vi "Log Monitor State Helper.vi"(6 "Laser ON?":bool, 7 "State Info":string, 8 "error in (no error)":errorcluster, 9 "Monitor":bool, 10 "STATUS.Ready":bool, 11 "EventLog in":refnum<class "EventLog.lvclass">) -> (0 "error out":errorcluster, 3 "EventLog out":refnum<class "EventLog.lvclass">)   [LabVIEW 2015, in "Tool Module.lvlib"]
uses:
  Tool Module.lvlib
  Event Logger Library/Event Log/EventLog.lvclass
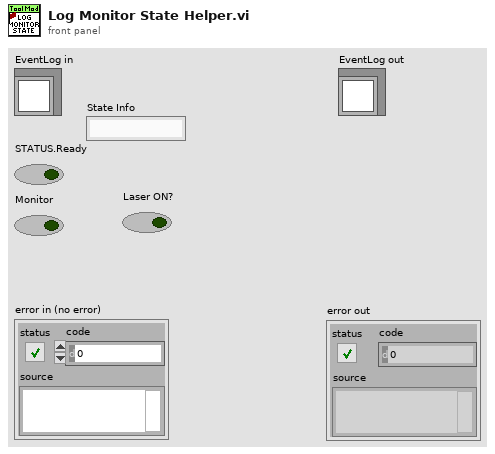
[diagram p1: front panel]
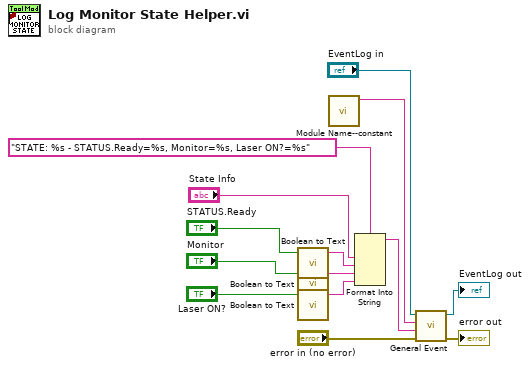
[diagram p0: block diagram]
diagram:
  n1 = call "Boolean to Text.vi"("selector"="STATUS.Ready") -> ("output string"=w12:string)  [unwired: 4 in]
  n2 = call "Boolean to Text.vi"("selector"="Monitor") -> ("output string"=w11:string)  [unwired: 4 in]
  n3 = call "Boolean to Text.vi"("selector"="Laser ON?") -> ("output string"=w8:string)  [unwired: 4 in]
  n4 = call "Module Name--constant.vi"() -> ("Module Name"=w1:string)  [unwired: 11 in]
  n5 = Format Into String(format string="STATE: %s - STATUS.Ready=%s, Monitor=%s, Laser ON?=%s", "State Info", w12, w11, w8) -> (resulting string=w6:string)  [unwired: 2 in, 1 out]
  n6 = call "General Event.vi"("error in (no error)"="error in (no error)", "Event Description"=w6, "Event Name"=w1, "EventLog ref"="EventLog in") -> ("error out"=→"error out":errorcluster, "EventLog ref"=→"EventLog out":refnum<class "EventLog.lvclass">)  [unwired: 6 in]
